vi "Event Structure - Each Button 1 A-Scan of Dataset for desired quantity.vi"() -> ()   [LabVIEW 2020]
panel:
  in  "Energy":bool
  in  "Peak Magnitude":bool
  in  "Peak Negative":bool
  in  "Peak Positive":bool
  out "Intensity Graph":dbl[][](graph)
  out "XY Graph":cluster{dbl[], dbl[]}(graph)
  out "output array":dbl[][](array[numeric])
  in  "Rows":dbl
  in  "Columns":dbl
  in  "Path":path=path "C:/Users/gaeta/Desktop/Unif Leerstof/Individual Project/Osc. Data/wetransfer-86c2d3/2DZXaxisscan 0.28MHz 30x30mm 20mvpp 1020L centre 390mm from td plane.mat"
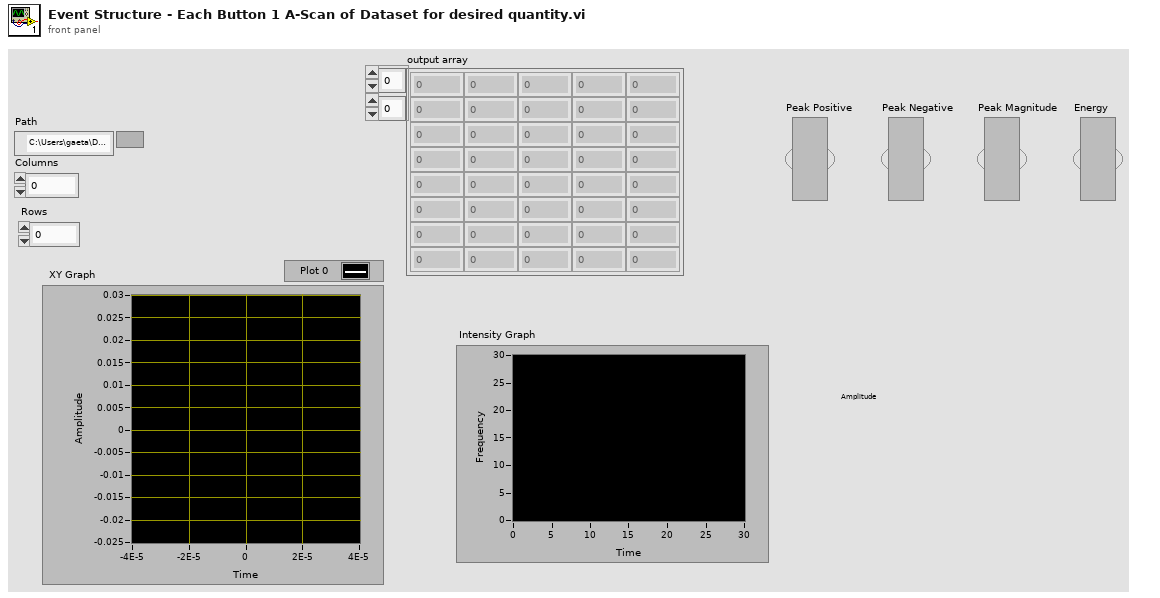
[diagram p1: front panel]
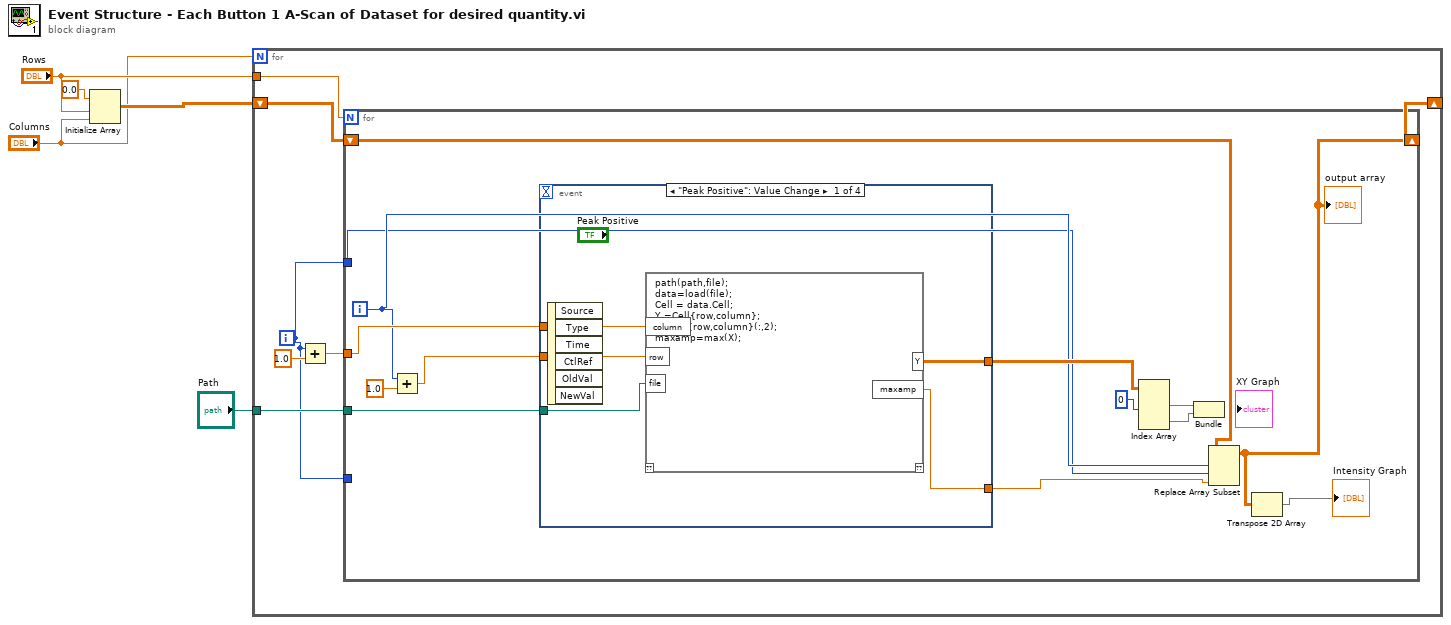
[diagram p0: block diagram]
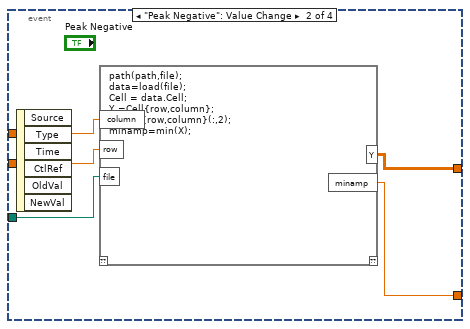
[diagram p2: hidden frame]
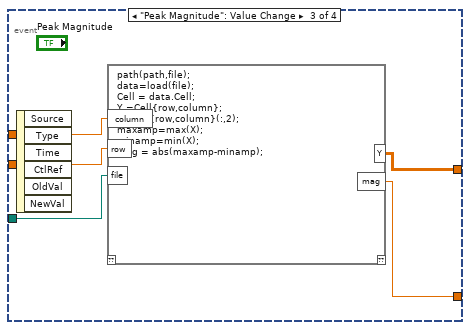
[diagram p3: hidden frame]
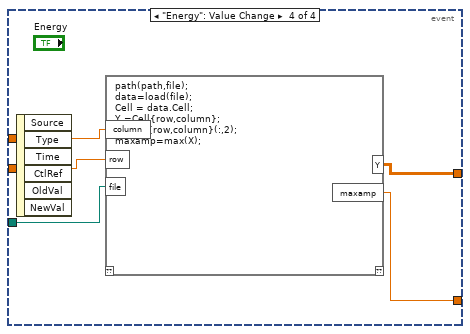
[diagram p4: hidden frame]
diagram:
  n1 = Initialize Array(0.0 ("element"), "Rows", "Columns") -> (w2:dbl[][])
  n2 = for {
    N: "Columns" -> [_]
    tunnel: "Path" -> [w12]
    tunnel: "Rows" -> [w10]
    shift-right: [w6] -> _
    shift-left: w2 -> [w9]
    i -> [w7]
    n3 = Add(x=w7, y=1.0) -> (x+y=w8:dbl)
    n4 = for {
      N: w10 -> [_]
      tunnel: w12 -> [w20]
      tunnel: w8 -> [w21]
      tunnel: w7 -> [_]
      shift-right: [w15] -> w6
      shift-left: w9 -> [w18]
      tunnel: w7 -> [w13]
      i -> [w17]
      n5 = Add(x=w17, y=1.0) -> (x+y=w22:dbl)
      n6 = event shown="[0] \"Peak Positive\": Value Change" {
        selector: _ -> [_ _ _ _]
        dyn-events: _ -> [_ _ _ _]
        timeout: _ -> [_ _ _ _]
        tunnel: w22 -> [w31 w32 w40 w45]
        tunnel: w21 -> [w30 w33 w41 w46]
        tunnel: w20 -> [w29 w36 w39 w44]
        tunnel: [w28 w35 w38 w43] -> w19
        tunnel: [w27 w34 w37 w42] -> w16
        event "Peak Positive": Value Change {
          n7 = event-data() -> ()  [unwired: 1 in, 6 out]
          n8 = script code="path(path,file);\ndata=load(file);\nCell = data.Cell;\nY =Cell{row,column};\nX=Cell{row,column}(:,2);\nmaxamp=max(X);"("row"=w31, "file"=w29, "column"=w30) -> ("Y"=w28:dbl[][], "maxamp"=w27:dbl)  [unwired: 1 in, 1 out]
        }
        event "Peak Negative": Value Change {
          n9 = event-data() -> ()  [unwired: 1 in, 6 out]
          n10 = script code="path(path,file);\ndata=load(file);\nCell = data.Cell;\nY =Cell{row,column};\nX=Cell{row,column}(:,2);\nminamp=min(X);"("row"=w32, "file"=w36, "column"=w33) -> ("Y"=w35:dbl[][], "minamp"=w34:dbl)  [unwired: 1 in, 1 out]
        }
        event "Peak Magnitude": Value Change {
          n11 = event-data() -> ()  [unwired: 1 in, 6 out]
          n12 = script code="path(path,file);\ndata=load(file);\nCell = data.Cell;\nY =Cell{row,column};\nX=Cell{row,column}(:,2);\nmaxamp=max(X);\nminamp=min(X);\nmag = abs(maxamp-minamp);"("row"=w40, "file"=w39, "column"=w41) -> ("Y"=w38:dbl[][], "mag"=w37:dbl)  [unwired: 1 in, 1 out]
        }
        event "Energy": Value Change {
          n13 = event-data() -> ()  [unwired: 1 in, 6 out]
          n14 = script code="path(path,file);\ndata=load(file);\nCell = data.Cell;\nY =Cell{row,column};\nX=Cell{row,column}(:,2);\nmaxamp=max(X);"("row"=w45, "file"=w44, "column"=w46) -> ("Y"=w43:dbl[][], "maxamp"=w42:dbl)  [unwired: 1 in, 1 out]
        }
      }
      n15 = Index Array(array=w19, index (col) #1=0 ("disabled index (col)")) -> (element #1=w24:dbl[], element #2=w25:dbl[])  [unwired: 3 in]
      n16 = Bundle(w24, w25) -> ()  [unwired: 1 in, 1 out]
      n17 = Replace Array Subset(array=w18, new element=w16, index (row)=w17, index (col)=w13) -> (w15:dbl[][])
      "output array" <- w15
      n18 = Transpose 2D Array(2D array=w15) -> (transposed array=→"Intensity Graph":dbl[][])
    }
  }
